vi "Add Exp.vi"(7 "Parameters":T1, 8 "error in (no error)":errorcluster, 9 "Exp name":string, 10 "Commentaires exp":string, 11 "Control-Client in":refnum<class "Control-Client.lvclass">) -> (0 "error out":errorcluster, 3 "Control-Client out":refnum<class "Control-Client.lvclass">)   [LabVIEW 2015, in "Control-Client.lvclass"]
uses:
  Control-Client.lvclass
  Experiments/Experiment.lvclass
  Control-Client.lvclass/Control-Client.ctl
  Experiments/Experiment.lvclass/Experiment.ctl
  Experiments/Experiments_group.lvclass/Experiments_group.ctl
  methods/Read Group #.vi
  Experiments/Experiments_group.lvclass
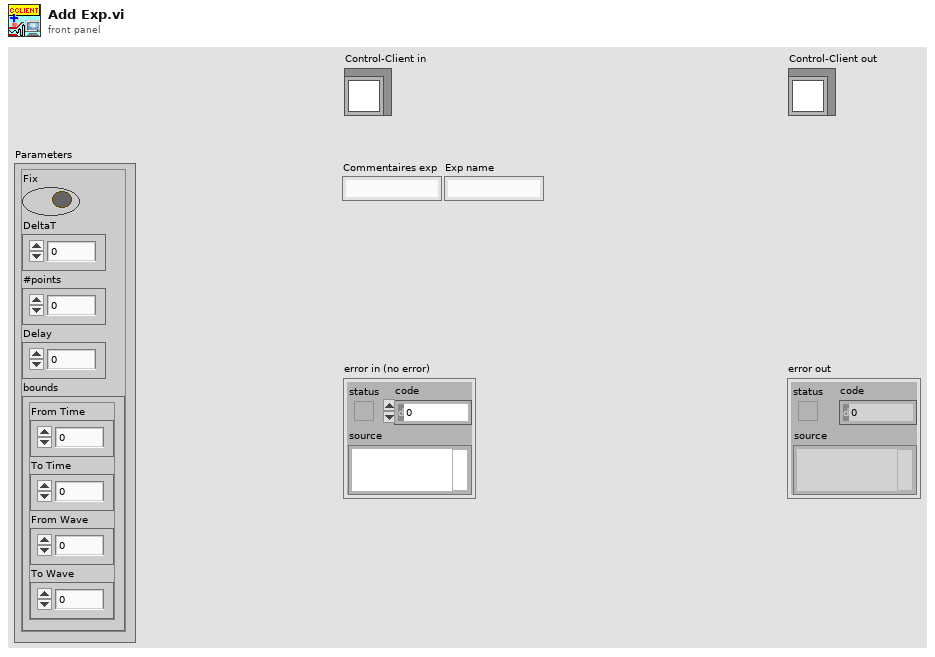
[diagram p1: front panel]
types:
  T1 = cluster{"Fix":bool, "DeltaT":dbl, "#points":i32, "Delay":dbl, "bounds":cluster{"From Time":dbl, "To Time":dbl, "From Wave":dbl, "To Wave":dbl}}
  T2 = typedef "Control-Client.lvclass/Delays-refs_CLIENT.ctl" = cluster{"# points":refnum<vi>, "Step, ps":refnum<vi>, "OZ, ps":refnum<vi>, "# current":refnum<vi>, "RDT, ps":refnum<vi>, "Total length, ps":refnum<vi>, "Kinetics length, ps":refnum<vi>, "Real zero, ps":refnum<vi>, "# par point":refnum<vi>}
  T3 = cluster{"From Time":dbl, "To Time":dbl, "From Wave":dbl, "To Wave":dbl}
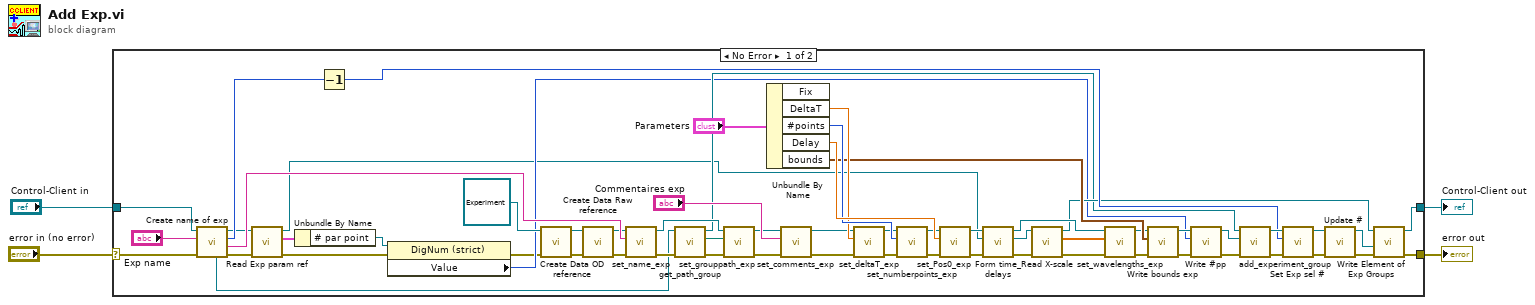
[diagram p0: block diagram]
diagram:
  n1 = case shown="No Error" "error in (no error)" {
    selector: "error in (no error)" -> [w34 w67]
    tunnel: [w46 w67] -> w3
    tunnel: [w47 w66] -> w1
    tunnel: "Control-Client in" -> [w21 w66]
    frame No Error {
      n2 = call "Create name of exp.vi"("error in (no error)"=w34, "Exp name"="Exp name", "Control-Client in"=w21) -> ("error out"=w7:errorcluster, "name out"=w65:string, "Numeric"=w57:i32, "Control-Client out"=w9:refnum<class "Control-Client.lvclass">, "Experiments_group out"=w19:refnum<class "Experiments_group.lvclass">)  [unwired: 4 in]
      n3 = call "Read Exp param ref.vi"("error in (no error)"=w7, "Control-Client in"=w9) -> ("error out"=w6:errorcluster, "Exp param ref"=w12:T2, "Control-Client out"=w8:refnum<class "Control-Client.lvclass">)  [unwired: 7 in]
      n4 = Unbundle By Name(w12) -> ("# par point"=w11:refnum<vi>)
      n5 = Decrement(x=w57) -> (x-1=w56:i32)
      n6 = property class="DigNum (strict)"(reference=w11, error in=w6) -> (error out=w5:errorcluster, "Value"=w10:i32)  [unwired: 1 out]
      n7 = call "Create Data OD reference.vi"("error in (no error)"=w5, "Experiment in"=refnum<class "Experiment.lvclass"> refnum ("Experiment.lvclass")) -> ("error out"=w23:errorcluster, "Experiment out"=w24:refnum<class "Experiment.lvclass">)  [unwired: 8 in]
      n8 = call "Create Data Raw reference.vi"("error in (no error)"=w23, "Experiment in"=w24) -> ("error out"=w26:errorcluster, "Experiment out"=w25:refnum<class "Experiment.lvclass">)  [unwired: 8 in]
      n9 = call "set_name_exp.vi"("error in (no error)"=w26, "Exp name"=w65, "Experiment.lvclass in"=w25) -> ("error out"=w54:errorcluster, "Experiment.lvclass out"=w55:refnum<class "Experiment.lvclass">)  [unwired: 7 in]
      n10 = call "get_path_group.vi"("error in (no error)"=w54, "Experiments_group.lvclass in"=w19) -> ("error out"=w61:errorcluster, "Path"=w53:path, "Experiments_group.lvclass out"=w17:refnum<class "Experiments_group.lvclass">)  [unwired: 7 in]
      n11 = call "set_grouppath_exp.vi"("error in (no error)"=w61, "GroupPath"=w53, "Experiment.lvclass in"=w55) -> ("error out"=w41:errorcluster, "Experiment.lvclass out"=w42:refnum<class "Experiment.lvclass">)  [unwired: 7 in]
      n12 = Unbundle By Name("Parameters") -> ("DeltaT"=w62:dbl, "#points"=w63:i32, "Delay"=w64:dbl, "bounds"=w31:T3)  [unwired: 1 out]
      n13 = call "set_comments_exp.vi"("error in (no error)"=w41, "Comments"="Commentaires exp", "Experiment.lvclass in"=w42) -> ("error out"=w45:errorcluster, "Experiment.lvclass out"=w44:refnum<class "Experiment.lvclass">)  [unwired: 7 in]
      n14 = call "set_deltaT_exp.vi"("error in (no error)"=w45, "deltaTlast"=w62, "Experiment.lvclass in"=w44) -> ("error out"=w38:errorcluster, "Experiment.lvclass out"=w40:refnum<class "Experiment.lvclass">)  [unwired: 6 in]
      n15 = call "set_numberpoints_exp.vi"("error in (no error)"=w38, "numberpoints"=w63, "Experiment.lvclass in"=w40) -> ("error out"=w39:errorcluster, "Experiment.lvclass out"=w37:refnum<class "Experiment.lvclass">)  [unwired: 6 in]
      n16 = call "set_Pos0_exp.vi"("error in (no error)"=w39, "Pos0,ps"=w64, "Experiment.lvclass in"=w37) -> ("error out"=w36:errorcluster, "Experiment.lvclass out"=w35:refnum<class "Experiment.lvclass">)  [unwired: 6 in]
      n17 = call "Form time_delays.vi"("error in (no error)"=w36, "Control-Client"=w8, "Experiment in"=w35) -> ("error out"=w27:errorcluster, "Control-Client out"=w18:refnum<class "Control-Client.lvclass">, "Experiment out"=w28:refnum<class "Experiment.lvclass">)  [unwired: 6 in]
      n18 = call "Read X-scale.vi"("error in (no error)"=w27, "Control-Client in"=w18) -> ("error out"=w33:errorcluster, "X-scale"=w32:dbl[], "Control-Client out"=w20:refnum<class "Control-Client.lvclass">)  [unwired: 7 in]
      n19 = call "set_wavelengths_exp.vi"("error in (no error)"=w33, "wavelengths"=w32, "Experiment.lvclass in"=w28) -> ("error out"=w30:errorcluster, "Experiment.lvclass out"=w29:refnum<class "Experiment.lvclass">)  [unwired: 7 in]
      n20 = call "Write bounds exp.vi"("error in (no error)"=w30, "Bounds"=w31, "Experiment in"=w29) -> ("error out"=w13:errorcluster, "Experiment out"=w16:refnum<class "Experiment.lvclass">)  [unwired: 7 in]
      n21 = call "Write #pp.vi"("error in (no error)"=w13, "#pp"=w10, "Experiment in"=w16) -> ("error out"=w14:errorcluster, "Experiment out"=w15:refnum<class "Experiment.lvclass">)  [unwired: 7 in]
      n22 = call-dynamic "add_experiment_group.vi"("error in (no error)"=w14, "Experiment.lvclass"=w15, "Experiments_group.lvclass in"=w17) -> ("error out"=w59:errorcluster, "Experiments_group.lvclass out"=w58:refnum<class "Experiments_group.lvclass">)  [unwired: 7 in]
      n23 = call "Set Exp sel #.vi"("error in (no error)"=w59, "Exp sel #"=w56, "Experiments_group in"=w58) -> ("error out"=w50:errorcluster, "Experiments_group out"=w51:refnum<class "Experiments_group.lvclass">)  [unwired: 7 in]
      n24 = call "Update #.vi"("error in (no error)"=w50, "Experiments_group in"=w51) -> ("error out"=w49:errorcluster, "Experiments_group out"=w48:refnum<class "Experiments_group.lvclass">)  [unwired: 8 in]
      n25 = call "Write Element of Exp Groups.vi"("error in (no error)"=w49, "Experiments_group.lvclass"=w48, "Control-Client in"=w20) -> ("error out"=w46:errorcluster, "Control-Client out"=w47:refnum<class "Control-Client.lvclass">)  [unwired: 7 in]
    }
    frame Error {
    }
  }
  "error out" <- w3
  "Control-Client out" <- w1
